vi "solar Ctrls Load.vi"(6 "ArrayDelimiters (1D,2D)":string[](array[string]), 7 "Section (\"\" = Use Target)":string, 8 "error in (no error)":errorcluster, 9 "Key Prefix (\"\")":string, 10 "Control Refnums":refnum<vi>[](array[refnum]), 11 "solar in":refnum<class "solar.lvclass">) -> (0 "error out":errorcluster, 3 "solar out":refnum<class "solar.lvclass">)   [LabVIEW 2018]
doc: "This VI loads the last saved control reference values from the temporary.ini file."
uses:
  cfg/solar_cfg Read File (Ref).vi
  solar.lvclass
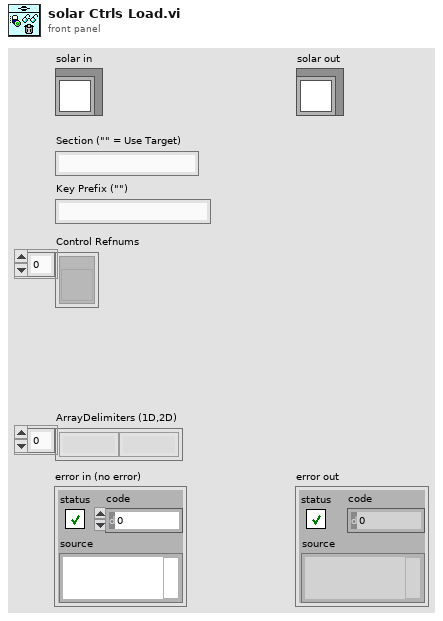
[diagram p1: front panel]
types:
  T1 = typedef "solar_app_ctl Info.ctl" = cluster{"AppName":string, "AppDir":path, "solar.ini":path, "ConfigsDir":path, "LogsDir":path, "CosmosDir":path, "ExePath":path, "vApp":string, "Part":string, "Setup":string, "Title":string, "Main.ini":path, "temp.ini":path, "vSOLAR":string, "Splash.png":string}
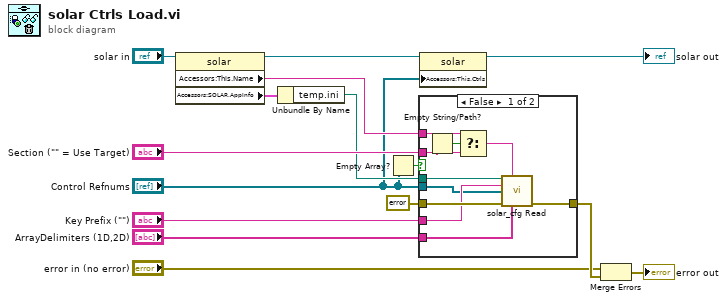
[diagram p0: block diagram]
diagram:
  n1 = property class="solar"(reference="solar in") -> (reference out=w8:refnum<class "solar.lvclass">, "Accessors:This.Name"=w5:string, "Accessors:SOLAR.AppInfo"=w7:T1)  [unwired: 1 in, 1 out]
  n2 = Unbundle By Name(w7) -> ("temp.ini"=w6:path)
  n3 = Empty Array?(array="Control Refnums") -> (empty?=w9:bool)
  n4 = case shown="False" w9 {
    tunnel: errorcluster {"status"=FALSE, "code"=0, "source"=""} ("error in (no error)") -> [w25 w26]
    tunnel: [w24 w26] -> w14
    tunnel: "Control Refnums" -> [w16 _]
    tunnel: "Key Prefix (\"\")" -> [w22 _]
    tunnel: w6 -> [w21 _]
    tunnel: "ArrayDelimiters (1D,2D)" -> [w23 _]
    tunnel: "Section (\"\" = Use Target)" -> [w18 _]
    tunnel: w5 -> [w17 _]
    frame False {
      n5 = Empty String/Path?(string/path=w18) -> (empty?=w20:bool)
      n6 = Select(t=w17, s=w20, f=w18) -> (s? t:f=w19:string)
      n7 = call-poly "solar_cfg Read.vi"("Config Path (*.ini)"=w21, "Section (\"\" = Use Filename)"=w19, "Key_Prefix (\"\")"=w22, "Ctrl Refnums"=w16, "error in (no error)"=w25, "ArrayDelimiters (1D,2D)"=w23) -> ("error out"=w24:errorcluster)  [unwired: 7 in, 2 out]
    }
    frame True {
    }
  }
  n8 = property class="solar"(reference=w8, "Accessors:This.Ctrls"="Control Refnums") -> (reference out=→"solar out":refnum<class "solar.lvclass">)  [unwired: 1 in, 1 out]
  n9 = Merge Errors("error in (no error)", w14) -> (→"error out":errorcluster)
